vi "fgv_Count error windows.vi"(8 "error in (no error)":errorcluster, 9 "Bounds of last error window":T1, 11 "Function":T2) -> (0 "error out":errorcluster, 1 "Bounds of last error window":T1, 3 "# of error windows open":i32)   [LabVIEW 2020]
uses:
  Error window positioning/Error window pos FGV states.ctl
  <vilib>/Utility/miscctls.llb/LVRectTypeDef.ctl
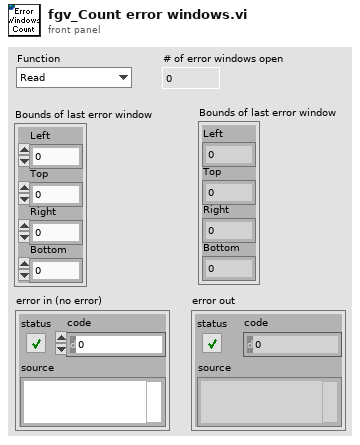
[diagram p1: front panel]
types:
  T1 = typedef "LVRectTypeDef.ctl" = cluster{"Left":i16, "Top":i16, "Right":i16, "Bottom":i16}
  T2 = typedef "Error window pos FGV states.ctl" = enum16{"Read", "Window closed", "Window opened", "Reset"}
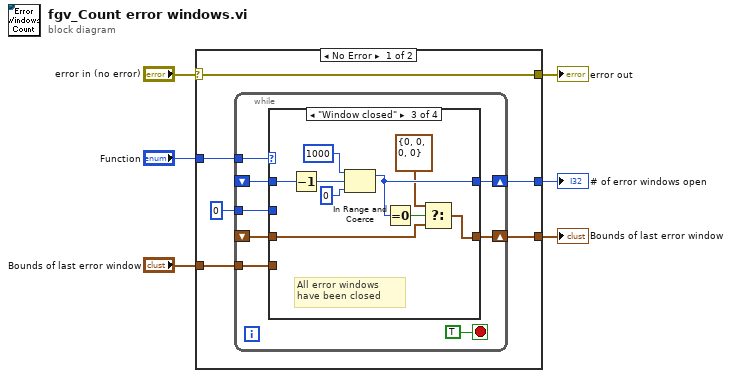
[diagram p0: block diagram]
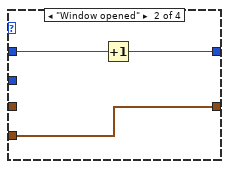
[diagram p3: hidden frame]
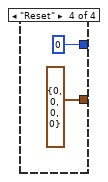
[diagram p4: hidden frame]
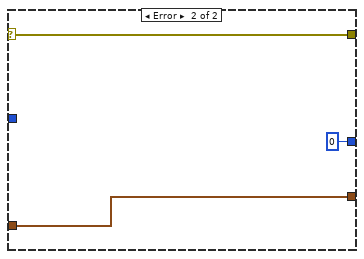
[diagram p5: hidden frame]
diagram:
  n1 = case shown="No Error" "error in (no error)" {
    selector: "error in (no error)" -> [w7 w39]
    tunnel: [w12 0] -> w6
    tunnel: "Function" -> [w11 _]
    tunnel: "Bounds of last error window" -> [w9 w37]
    tunnel: [w8 w37] -> w3
    tunnel: [w7 w39] -> w1
    frame No Error {
      n2 = while {
        tunnel: 0 -> [w18]
        shift-right: [w17] -> w12
        shift-left: _ -> [w19]
        tunnel: w11 -> [w16]
        tunnel: w9 -> [w15]
        shift-right: [w14] -> w8
        shift-left: _ -> [w13]
        stop <- TRUE stop-if-true
        n3 = case shown="\"Window closed\"" w16 {
          tunnel: w19 -> [w22 w25 w34 _]
          tunnel: w18 -> [_ _ _ _]
          tunnel: [w22 w23 w30 0] -> w17
          tunnel: w15 -> [_ w24 _ _]
          tunnel: [w21 w24 w28 T1 {"Left"=0, "Top"=0, "Right"=0, "Bottom"=0} ("Bounds of last error window")] -> w14
          tunnel: w13 -> [w21 _ w26 _]
          frame "Read", Default {
          }
          frame "Window opened" {
            n4 = Increment(x=w25) -> (x+1=w23:i32)
          }
          frame "Window closed" {
            # "All error windows have been closed"
            n5 = Decrement(x=w34) -> (x-1=w31:i32)
            n6 = In Range and Coerce(upper limit=1000, x=w31, lower limit=0) -> (coerced(x)=w30:i32)  [unwired: 1 out]
            n7 = Equal To 0?(x=w30) -> (x = 0?=w29:bool)
            n8 = Select(t=T1 {"Left"=0, "Top"=0, "Right"=0, "Bottom"=0}, s=w29, f=w26) -> (s? t:f=w28:T1)
          }
          frame "Reset" {
          }
        }
      }
    }
    frame Error {
    }
  }
  "# of error windows open" <- w6
  "error out" <- w1
  "Bounds of last error window" <- w3
